vi "Configure Gate Coupling.vi"(5 "Coupling Type (T: Enable)":bool=TRUE, 6 "Coupling Shape (T: Enable)":bool=TRUE, 7 "Coupling State (F: Disable)":bool, 8 "error in (no error)":errorcluster, 9 "Coupling Stimulus (T: Enable)":bool=TRUE, 10 "Channel (1)":i32=1, 11 "VISA resource name":refnum<visa-resource-name>) -> (0 "error out":errorcluster, 3 "VISA resource name out":refnum<visa-resource-name>)   [LabVIEW 2018, in "Keysight PNA Series.lvlib"]
doc: "Configures the time domain gating parameters to be coupled."
uses:
  Keysight PNA Series.lvlib
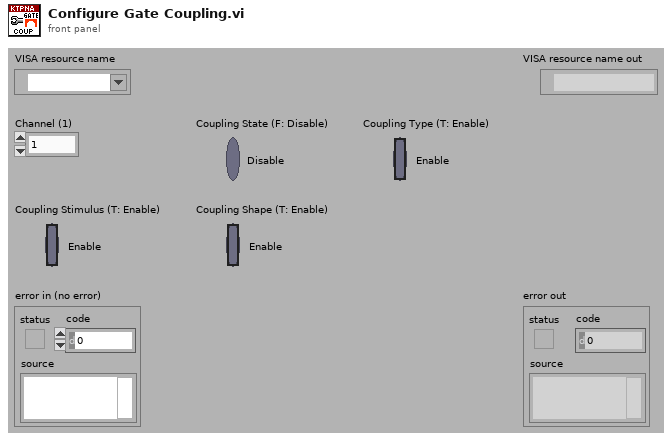
[diagram p1: front panel]
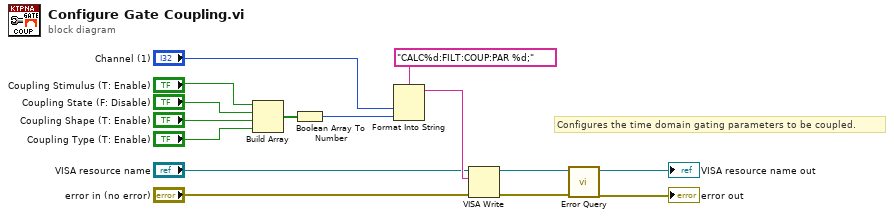
[diagram p0: block diagram]
diagram:
  # "Configures the time domain gating parameters to be coupled."
  n1 = Build Array("Coupling Stimulus (T: Enable)", "Coupling State (F: Disable)", "Coupling Shape (T: Enable)", "Coupling Type (T: Enable)") -> (w2:bool[])
  n2 = Boolean Array To Number(Boolean array=w2) -> (number=w1:u32)
  n3 = Format Into String(format string="CALC%d:FILT:COUP:PAR %d;", "Channel (1)", w1) -> (resulting string=w13:string)  [unwired: 2 in, 1 out]
  n4 = VISA Write(VISA resource name="VISA resource name", write buffer=w13, error in (no error)="error in (no error)") -> (VISA resource name out=w10:refnum<visa-resource-name>, error out=w9:errorcluster)  [unwired: 1 out]
  n5 = call "Error Query.vi"("error in (no error)"=w9, "VISA resource name"=w10) -> ("error out"=→"error out":errorcluster, "VISA resource name out"=→"VISA resource name out":refnum<visa-resource-name>)  [unwired: 6 in, 2 out]
